vi "Configure Null Offset.vi"(7 "Enable Offset (T: Enable)":bool=TRUE, 8 "error in (no error)":errorcluster, 9 "Manual Offset (0)":dbl, 10 "Offset Mode (0: First Reading)":u16(ring) items=["First Reading", "Manual Offset"], 11 "VISA resource name":refnum<visa-resource-name>) -> (0 "error out":errorcluster, 3 "VISA resource name out":refnum<visa-resource-name>)   [LabVIEW 2012, in "Keithley 24XX.lvlib"]
doc: "Configures the null offset settings for limit testing."
uses:
  <instrlib>/Keithley 24XX/Keithley 24XX.lvlib
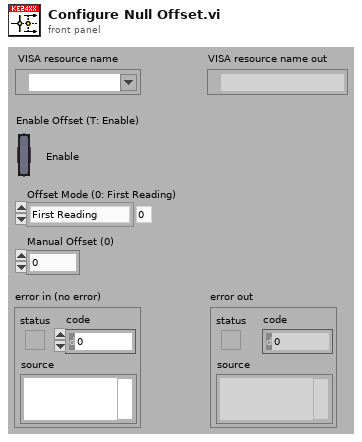
[diagram p1: front panel]
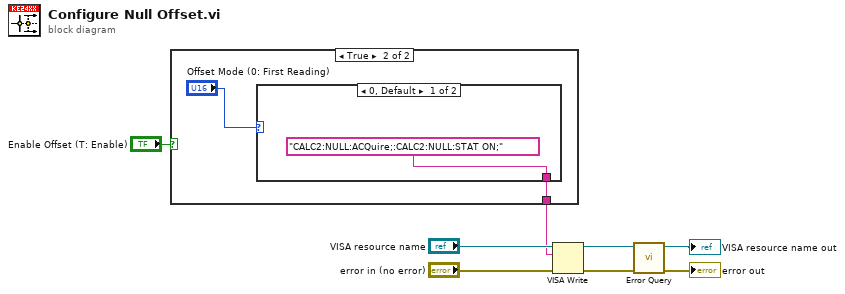
[diagram p0: block diagram]
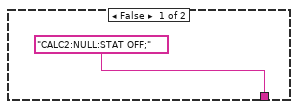
[diagram p2: hidden frame]
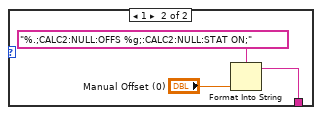
[diagram p3: hidden frame]
diagram:
  n1 = case shown="True" "Enable Offset (T: Enable)" {
    tunnel: ["CALC2:NULL:STAT OFF;" w11] -> w2
    frame False {
    }
    frame True {
      n2 = case shown="0, Default" "Offset Mode (0: First Reading)" {
        tunnel: ["CALC2:NULL:ACQuire;:CALC2:NULL:STAT ON;" w15] -> w11
        frame 0, Default {
        }
        frame 1 {
          n3 = Format Into String(format string="%.;CALC2:NULL:OFFS %g;:CALC2:NULL:STAT ON;", "Manual Offset (0)") -> (resulting string=w15:string)  [unwired: 2 in, 1 out]
        }
      }
    }
  }
  n4 = VISA Write(VISA resource name="VISA resource name", write buffer=w2, error in (no error)="error in (no error)") -> (VISA resource name out=w6:refnum<visa-resource-name>, error out=w3:errorcluster)  [unwired: 1 out]
  n5 = call <instrlib>:"Error Query.vi"("error in (no error)"=w3, "VISA resource name"=w6) -> ("error out"=→"error out":errorcluster, "VISA resource name out"=→"VISA resource name out":refnum<visa-resource-name>)  [unwired: 6 in, 2 out]
